vi "Cached_Build.vi"(8 "error in (no error)":errorcluster, 11 "AB_Build in":refnum<class "AB_Build.lvclass">) -> (0 "error out":errorcluster, 1 "Dependencies":T1[](array[typedef]), 2 "valid?":bool, 3 "AB_Build out":refnum<class "AB_Build.lvclass">, 4 "GeneratedFileGUIDs":string[](array[string]))   [LabVIEW 2020, in "AB_Build.lvclass"]
uses:
  <vilib>/AppBuilder/AB_Classes/Build/AB_Build.lvclass
  <vilib>/AppBuilder/AB_Dependency.ctl
  <vilib>/Utility/lvfile.llb/LVFileType.ctl
  <vilib>/AppBuilder/AB_Classes/Build/AB_Build.lvclass/AB_Build.ctl
  <resource>/Framework/Providers/Common/provcom_StringGlobals.vi
  <vilib>/Utility/lvfile.llb/NI_FileType.lvlib
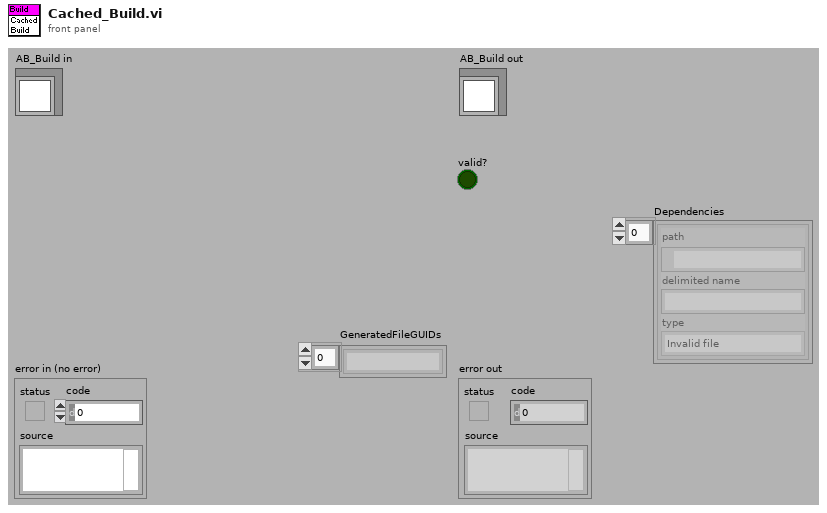
[diagram p1: front panel]
types:
  T1 = typedef "AB_Dependency.ctl" = cluster{"path":path, "delimited name":string, "type":T2}
  T2 = typedef "NI_FileType.lvlib/LVFileType.ctl" = enum32{"Invalid file", "Unknown type", "Instrument", "Control", "Polymorphic VI", "Project", "Library", "LVClass", "XControl", "XNode", "Shared library", ".NET assembly", "ActiveX interface", "CIN", "Run-time menu", "Palette menu", "Help file", "LLB", "XNode Edit Dependency", "Class Private Data Control", "Statechart", "MathScript .m file", "Ladder Diagram", "LVLibp", "XNode Build Dependency"}
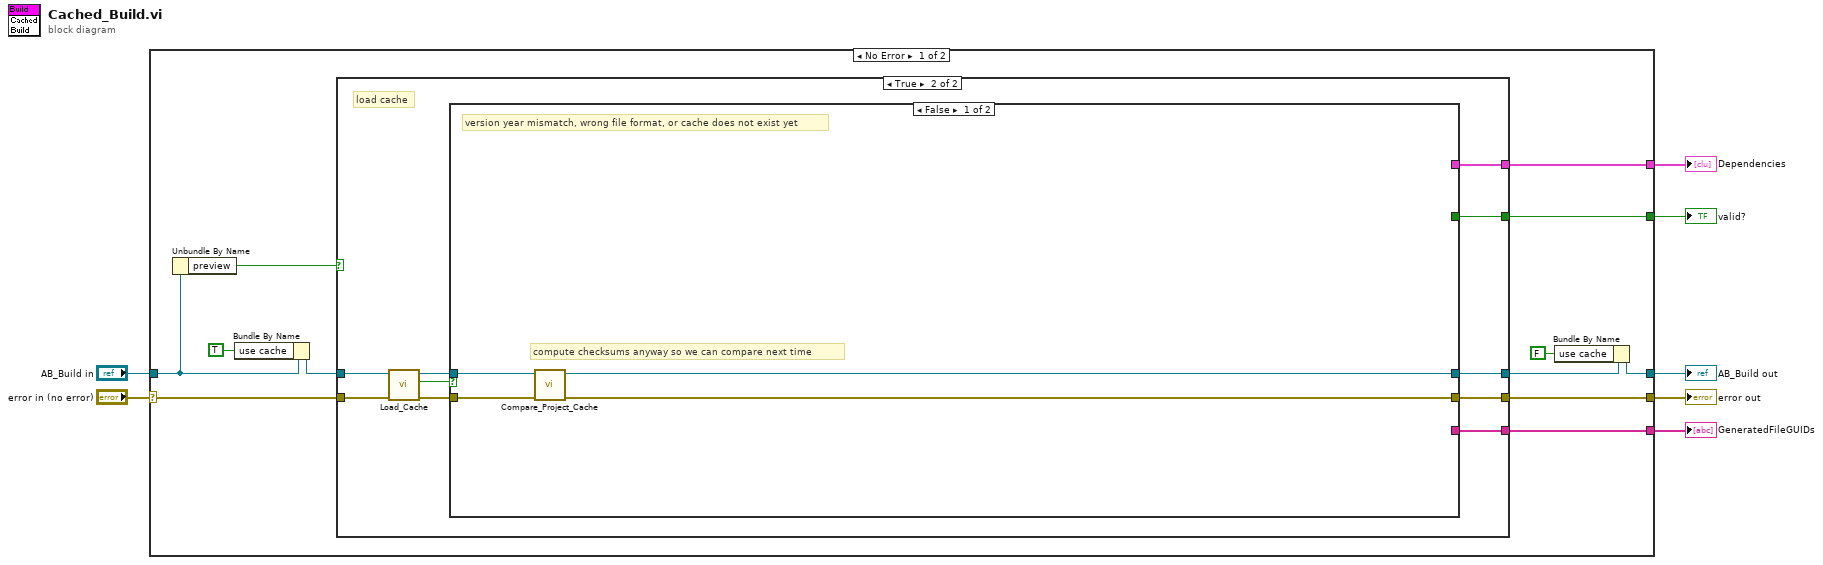
[diagram p0: block diagram]
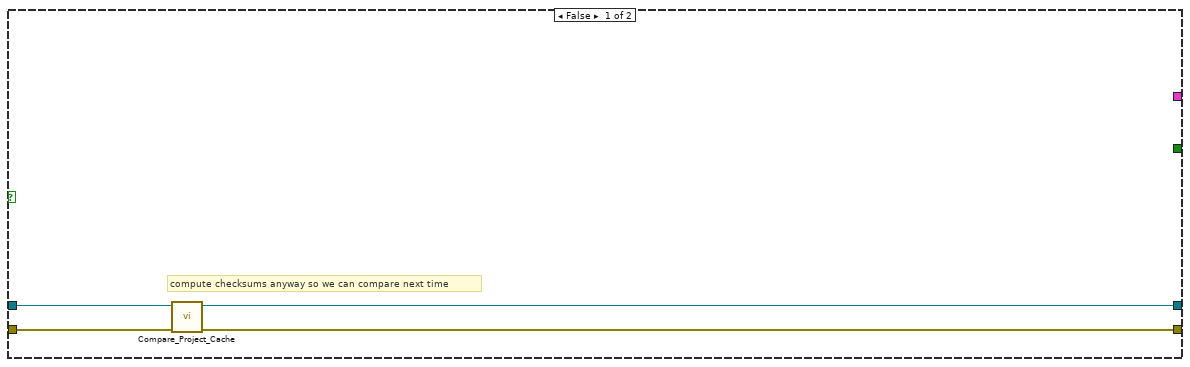
[diagram p2: hidden frame]
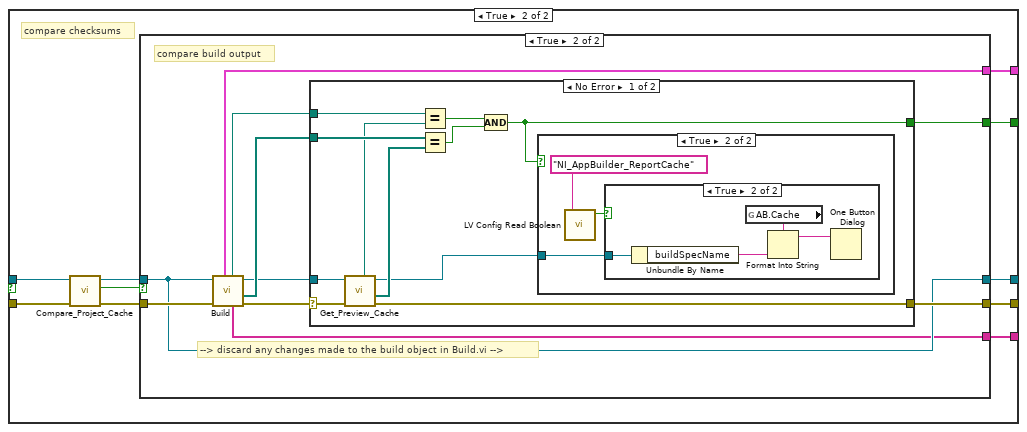
[diagram p3: hidden frame]
diagram:
  n1 = case shown="No Error" "error in (no error)" {
    selector: "error in (no error)" -> [w19 w80]
    tunnel: [w18 w80] -> w6
    tunnel: [w16 w79] -> w4
    tunnel: "AB_Build in" -> [w12 w79]
    tunnel: [w17 _] -> w3
    tunnel: [w9 _] -> w2
    tunnel: [w8 _] -> w1
    frame No Error {
      n2 = Unbundle By Name(w12) -> ("preview"=w10:bool)
      n3 = Bundle By Name(cluster=w12, "use cache"=TRUE ("use cache?")) -> (w11:refnum<class "AB_Build.lvclass">)
      n4 = case shown="True" w10 {
        tunnel: [w20 w33] -> w18
        tunnel: w19 -> [w21 w27]
        tunnel: [w22 w32] -> w15
        tunnel: w11 -> [w23 w28]
        tunnel: [_ w31] -> w17
        tunnel: [_ w26] -> w9
        tunnel: [_ w25] -> w8
        frame False {
          # "compute checksums anyway so we can compare next time"
          n5 = call <vilib>:"Compare_Project_Cache.vi"("error in (no error)"=w21, "AB_Build in"=w23) -> ("error out"=w20:errorcluster, "AB_Build out"=w22:refnum<class "AB_Build.lvclass">)  [unwired: 7 in, 1 out]
        }
        frame True {
          # "load cache"
          n6 = call <vilib>:"Load_Cache.vi"("error in (no error)"=w27, "AB_Build in"=w28) -> ("error out"=w29:errorcluster, "valid format?"=w24:bool, "AB_Build out"=w30:refnum<class "AB_Build.lvclass">)  [unwired: 7 in]
          n7 = case shown="False" w24 {
            tunnel: [w34 w46] -> w33
            tunnel: [w36 w44] -> w32
            tunnel: [_ w42] -> w31
            tunnel: w30 -> [w37 w41]
            tunnel: w29 -> [w35 w40]
            tunnel: [_ w39] -> w26
            tunnel: [_ w38] -> w25
            frame False {
              # "compute checksums anyway so we can compare next time"
              # "version year mismatch, wrong file format, or cache does not exist yet"
              n8 = call <vilib>:"Compare_Project_Cache.vi"("error in (no error)"=w35, "AB_Build in"=w37) -> ("error out"=w34:errorcluster, "AB_Build out"=w36:refnum<class "AB_Build.lvclass">)  [unwired: 7 in, 1 out]
            }
            frame True {
              # "compare checksums"
              n9 = call <vilib>:"Compare_Project_Cache.vi"("error in (no error)"=w40, "AB_Build in"=w41) -> ("error out"=w47:errorcluster, "valid?"=w43:bool, "AB_Build out"=w45:refnum<class "AB_Build.lvclass">)  [unwired: 7 in]
              n10 = case shown="True" w43 {
                tunnel: w47 -> [w48 w59]
                tunnel: [w48 w54] -> w46
                tunnel: w45 -> [w49 w53]
                tunnel: [w49 w53] -> w44
                tunnel: [_ w57] -> w42
                tunnel: [_ w51] -> w39
                tunnel: [_ w50] -> w38
                frame False {
                }
                frame True {
                  # "--> discard any changes made to the build object in Build.vi -->"
                  # "compare build output"
                  n11 = call-dynamic "Build.vi"("error in (no error)"=w59, "Build in"=w53) -> ("error out"=w55:errorcluster, "GeneratedFiles"=w56:path[], "Build out"=w52:refnum<class "AB_Build.lvclass">, "GeneratedFileGUIDs"=w50:string[], "OutputDirectory"=w58:path, "Dependencies"=w51:T1[])  [unwired: 3 in, 1 out]
                  n12 = case shown="No Error" w55 {
                    selector: w55 -> [w64 w78]
                    tunnel: w52 -> [w66 _]
                    tunnel: w58 -> [w70 _]
                    tunnel: [w61 _] -> w57
                    tunnel: w56 -> [w67 _]
                    tunnel: [w63 w78] -> w54
                    frame No Error {
                      n13 = call <vilib>:"Get_Preview_Cache.vi"("error in (no error)"=w64, "AB_Build in"=w66) -> ("error out"=w63:errorcluster, "GeneratedFiles"=w62:path[], "AB_Build out"=w60:refnum<class "AB_Build.lvclass">, "OutputDirectory"=w65:path)  [unwired: 6 in]
                      n14 = Equal?(x=w70, y=w65) -> (x = y?=w69:bool)
                      n15 = Equal?(x=w67, y=w62) -> (x = y?=w68:bool)
                      n16 = Compound Arithmetic op=AND(w69, w68) -> (w61:bool)
                      n17 = case shown="True" w61 {
                        tunnel: w60 -> [_ w72]
                        frame False {
                        }
                        frame True {
                          n18 = call <resource>:"LV Config Read Boolean.vi"("key"="NI_AppBuilder_ReportCache") -> ("value"=w73:bool)  [unwired: 2 in, 4 out]
                          n19 = case shown="True" w73 {
                            tunnel: w72 -> [_ w75]
                            frame False {
                            }
                            frame True {
                              n20 = Unbundle By Name(w75) -> ("buildSpecName"=w74:string)
                              n21 = global read "provcom_StringGlobals.vi" "AB.Cache"() -> (w77:string)
                              n22 = Format Into String(format string=w77, w74) -> (resulting string=w76:string)  [unwired: 2 in, 1 out]
                              n23 = One Button Dialog(message=w76) -> ()  [unwired: 1 in, 1 out]
                            }
                          }
                        }
                      }
                    }
                    frame Error {
                    }
                  }
                }
              }
            }
          }
        }
      }
      n24 = Bundle By Name(cluster=w15, "use cache"=FALSE) -> (w16:refnum<class "AB_Build.lvclass">)
    }
    frame Error {
    }
  }
  "error out" <- w6
  "AB_Build out" <- w4
  "valid?" <- w3
  "Dependencies" <- w2
  "GeneratedFileGUIDs" <- w1
